vi "Example Callback.vi"() -> ()   [LabVIEW 2010]
uses:
  C:/tf/play/labview/Tinkerforge.dll
  Tinkerforge.dll
panel:
  out "period":i64
  out "altitude (m)":sgl format="%#_13g"
  in  "stop":bool
  out "air pressure (mbar)":sgl format="%#_13g"
  in  "uid":string="jmQ"
  in  "port":i32=4223
  in  "host":string="localhost"
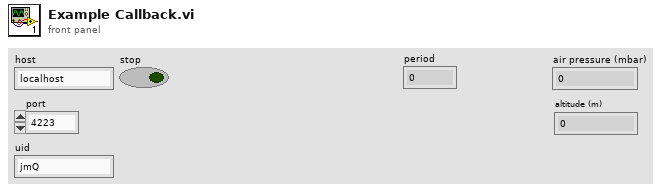
[diagram p1: front panel]
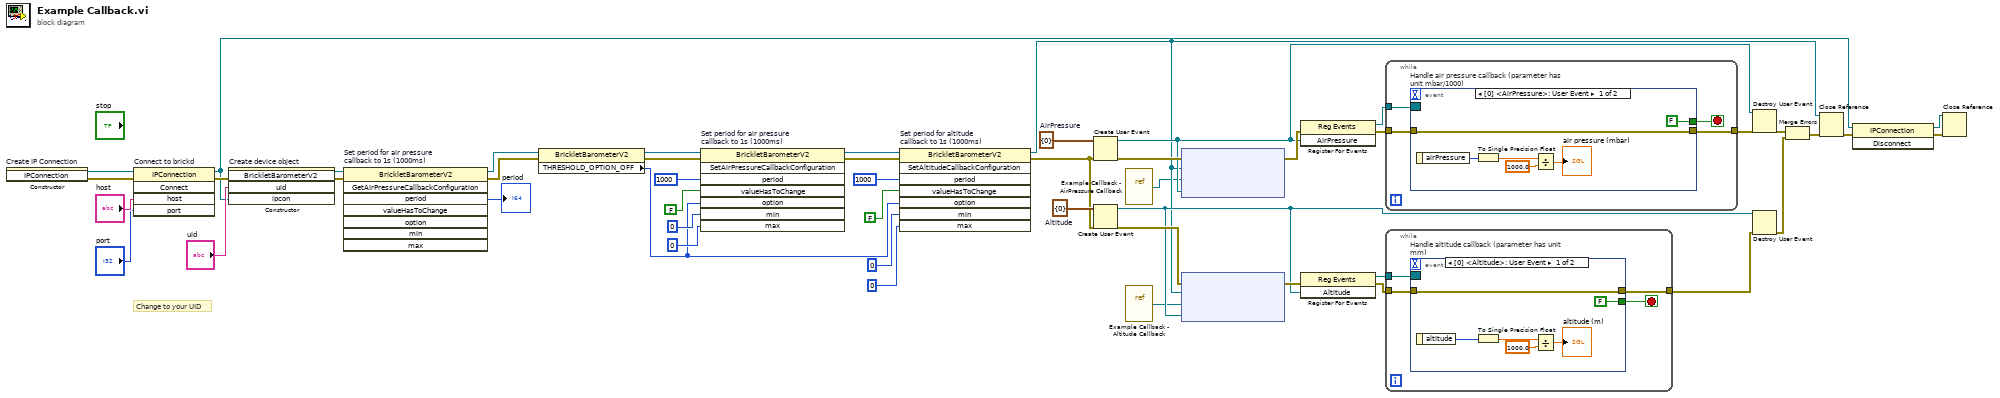
[diagram p0: block diagram]
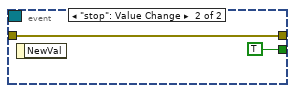
[diagram p2: hidden frame]
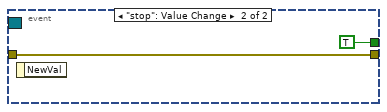
[diagram p3: hidden frame]
diagram:
  w25 = cluster{"altitude":i32} {"altitude"=0}  # Altitude
  w34 = cluster{"airPressure":i32} {"airPressure"=0}  # AirPressure
  # "Change to your UID"
  n1 = constructor on="Create IP Connection" class="IPConnection"() -> (reference out=w49:refnum<k24>, error out=w17:errorcluster)  [unwired: 3 in, 1 out]
  n2 = invoke on="Connect to brickd" class="IPConnection" method="Connect"(reference=w49, error in=w17, "host"="host", "port"="port") -> (reference out=w42:refnum<k24>, error out=w45:errorcluster)  [unwired: 1 in, 3 out]
  n3 = constructor on="Create device object" class="BrickletBarometerV2"(error in=w45, "uid"="uid", "ipcon"=w42) -> (reference out=w7:refnum<k24>, error out=w5:errorcluster)  [unwired: 2 in, 3 out]
  n4 = invoke on="Set period for air pressure\ncallback to 1s (1000ms)" class="BrickletBarometerV2" method="GetAirPressureCallbackConfiguration"(reference=w7, error in=w5) -> (reference out=w6:refnum<k24>, error out=w4:errorcluster, "period"=→"period":i64)  [unwired: 6 in, 5 out]
  n5 = property class="BrickletBarometerV2"(reference=w6, error in=w4) -> (reference out=w9:refnum<k24>, error out=w10:errorcluster, "THRESHOLD_OPTION_OFF"=w8:u16)
  n6 = invoke on="Set period for air pressure\ncallback to 1s (1000ms)" class="BrickletBarometerV2" method="SetAirPressureCallbackConfiguration"(reference=w9, error in=w10, "period"=i64 1000, "valueHasToChange"=FALSE, "option"=w8, "min"=0, "max"=0) -> (reference out=w18:refnum<k24>, error out=w19:errorcluster)  [unwired: 1 in, 6 out]
  n7 = invoke on="Set period for altitude\ncallback to 1s (1000ms)" class="BrickletBarometerV2" method="SetAltitudeCallbackConfiguration"(reference=w18, error in=w19, "period"=i64 1000, "valueHasToChange"=FALSE, "option"=w8, "min"=0, "max"=0) -> (reference out=w26:refnum<k24>, error out=w24:errorcluster)  [unwired: 1 in, 6 out]
  n8 = Create User Event(user event datatype=w34, error in=w24) -> (user event=w35:refnum<user-event>, error out=w40:errorcluster)
  n9 = Create User Event(user event datatype=w25, error in=w24) -> (user event=w27:refnum<user-event>, error out=w32:errorcluster)
  n10 = vi-ref "Example Callback - AirPressure Callback.vi"() -> ("vi reference"=w2:refnum<vi>)
  n11 = vi-ref "Example Callback - Altitude Callback.vi"() -> ("vi reference"=w1:refnum<vi>)
  n12 = node ("Register Event Callback")(w40, w26, w2, w35) -> (w39:errorcluster)  [unwired: 1 in, 1 out]
  n13 = node ("Register Event Callback")(w32, w26, w1, w27) -> (w31:errorcluster)  [unwired: 1 in, 1 out]
  n14 = register-events(error in=w39, w35) -> (reference out=w38:refnum<event-registration>, error out=w36:errorcluster)  [unwired: 1 in]
  n15 = register-events(error in=w31, w27) -> (reference out=w30:refnum<event-registration>, error out=w28:errorcluster)  [unwired: 1 in]
  n16 = while {
    tunnel: w38 -> [w53]
    tunnel: [w52] -> w37
    tunnel: w36 -> [w51]
    stop <- w50 stop-if-true
    n17 = event "Handle air pressure callback (parameter has unit mbar/1000)" shown="[0] <AirPressure>: User Event" {
      selector: w53 -> [_ _]
      dyn-events: _ -> [_ _]
      timeout: _ -> [_ _]
      tunnel: [w56 w60] -> w52
      tunnel: w51 -> [w56 w60]
      tunnel: [FALSE TRUE] -> w50
      event User Event {
        n18 = event-data() -> ("airPressure"=w57:i32)  [unwired: 1 in]
        n19 = To Single Precision Float(number=w57) -> (single precision float=w58:sgl)
        n20 = Divide(x=w58, y=sgl 1000.0) -> (x/y=→"air pressure (mbar)":sgl)
      }
      event "stop": Value Change {
        n21 = event-data() -> ()  [unwired: 1 in, 1 out]
      }
    }
  }
  n22 = while {
    tunnel: w30 -> [w65]
    tunnel: [w64] -> w29
    tunnel: w28 -> [w63]
    stop <- w62 stop-if-true
    n23 = event "Handle altitude callback (parameter has unit mm)" shown="[0] <Altitude>: User Event" {
      selector: w65 -> [_ _]
      dyn-events: _ -> [_ _]
      timeout: _ -> [_ _]
      tunnel: [w68 w72] -> w64
      tunnel: w63 -> [w68 w72]
      tunnel: [FALSE TRUE] -> w62
      event User Event {
        n24 = event-data() -> ("altitude"=w69:i32)  [unwired: 1 in]
        n25 = To Single Precision Float(number=w69) -> (single precision float=w70:sgl)
        n26 = Divide(x=w70, y=sgl 1000.0) -> (x/y=→"altitude (m)":sgl)
      }
      event "stop": Value Change {
        n27 = event-data() -> ()  [unwired: 1 in, 1 out]
      }
    }
  }
  n28 = Destroy User Event(user event=w35, error in=w37) -> (error out=w22:errorcluster)
  n29 = Destroy User Event(user event=w27, error in=w29) -> (error out=w23:errorcluster)
  n30 = Merge Errors(w22, w23) -> (w21:errorcluster)
  n31 = Close Reference(reference=w26, error in (no error)=w21) -> (error out=w44:errorcluster)
  n32 = invoke class="IPConnection" method="Disconnect"(reference=w42, error in=w44) -> (reference out=w41:refnum<k24>, error out=w43:errorcluster)  [unwired: 1 in, 1 out]
  n33 = Close Reference(reference=w41, error in (no error)=w43) -> ()  [unwired: 1 out]
